vi "Process.vi"(8 "error in":errorcluster, 11 "SystemController":refnum<class "SystemController.lvclass">) -> (0 "error out":errorcluster, 3 "SystemController out":refnum<class "SystemController.lvclass">)   [LabVIEW 2017, in "SystemController.lvclass"]
doc: "---------------------------------------------------------------\nJKI State Machine Objects™\nhttp://jki.net/state-machine-objects/\nCopyright (C) 2005-2015, JKI <info@jki.net>\nALL RIGHTS RESERVEDJKI State Machine Objects (SMO) 1.0.0.5\nJKI - JKI\nCopyright (c) 2016, JKI"
uses:
  SystemController.lvclass
  C:/Program Files (x86)/National Instruments/LabVIEW 2017/vi.lib/JKI/JKI SMO/SMO/SMO.lvclass
  <vilib>/JKI/JKI SMO/SMO/Typedefs/Parent Call--Enum.ctl
  ImageFacialDetection_class/FindFaces_IMAQ.vi
  ImageFacialDetection_class/FindEyes_IMAQ.vi
  <vilib>/JKI/JKI SMO/SMO/SMO.lvclass
  Camera/Camera_class/Camera.lvclass
  ImageFacialDetection_class/ImageFacialDetection.lvclass
panel:
  out "Image":T1(plugin-control)
  out "Connected":bool
  # "For instructions on how to use the JKI State Machine Objects, examples and video tutorials, visit:\nhttp://jki.net/state-machine-objects/\n\nJKI State Machine Objects™\nhttp://jki.net/state-machine-objects/\nCopyright (C) 2005-2015, JKI <info@jki.net>\nALL RIGHTS RESERVED"
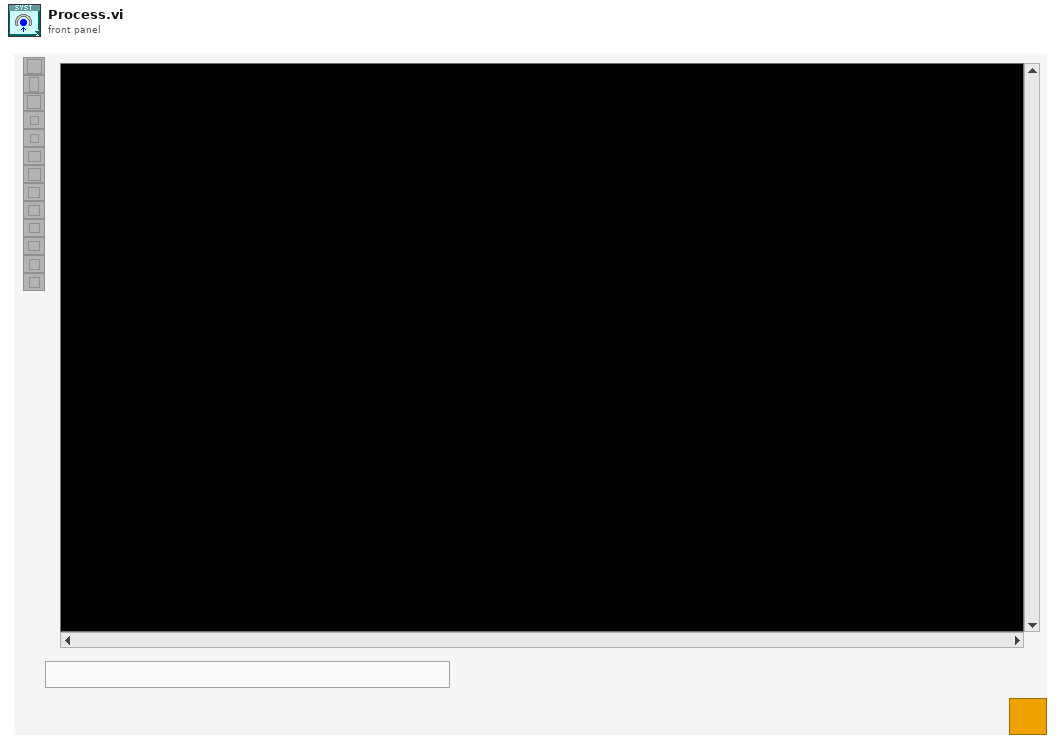
[diagram p1: front panel]
types:
  T1 = typedef "IMAQ Image.ctl" = refnum<image>
  T2 = typedef "SMO.lvclass/Parent Call--Enum.ctl" = enum16{"Allows parent to run", "Does not request parent to run"}
  T3 = enum32{"invalid app kind", "Development System", "Run Time System", "Student Edition", "Embedded LabVIEW", "Evaluation", "Custom"}
  T4 = enum32{"Invalid", "Standard", "Closed", "Hidden", "Minimized", "Maximized"}
  T5 = typedef "SystemController.lvclass/Configuration--Cluster.ctl" = cluster{"Camera":T6, "Find Eyes":bool, "Acquisition Rate (ms)":i32, "Image Buffer Length":i32}
  T6 = typedef "SystemController.lvclass/CameraConfig--Cluster.ctl" = cluster{"Simulate Camera":bool, "IMAQ Camera":T7, "Simulated Image Folder":path}
  T7 = typedef "Camera_IMAQdx.lvclass/Configuration--Cluster.ctl" = cluster{"Camera Interface Name":string, "Number of Buffers":u32, "Image Name":string, "Image Type":T8}
  T8 = typedef "Image Type" = u32
  T9 = typedef "SystemController.lvclass/Dependencies--Cluster.ctl" = cluster{"Camera":refnum<class "Camera.lvclass">, "ImageFacialDetection":refnum<class "ImageFacialDetection.lvclass">}
  T10 = cluster{"Core":cluster{"Current VI Reference":refnum<vi>, "Close Panel on Exit?":bool, "error":errorcluster}, "Self Reference":refnum<class "SystemController.lvclass">, "Dependencies":T9, "Find Eyes":bool, "Camera Connected":bool, "New Image":T1}
  T11 = cluster{"Current VI Reference":refnum<vi>, "Close Panel on Exit?":bool, "error":errorcluster}
  T12 = typedef "SMO.lvclass/Protected Events.ctl" = cluster{"StopProcesses":refnum<user-event>, "AbortProcesses":refnum<user-event>, "Config Changed":refnum<user-event>, "Dependency":refnum<user-event>}
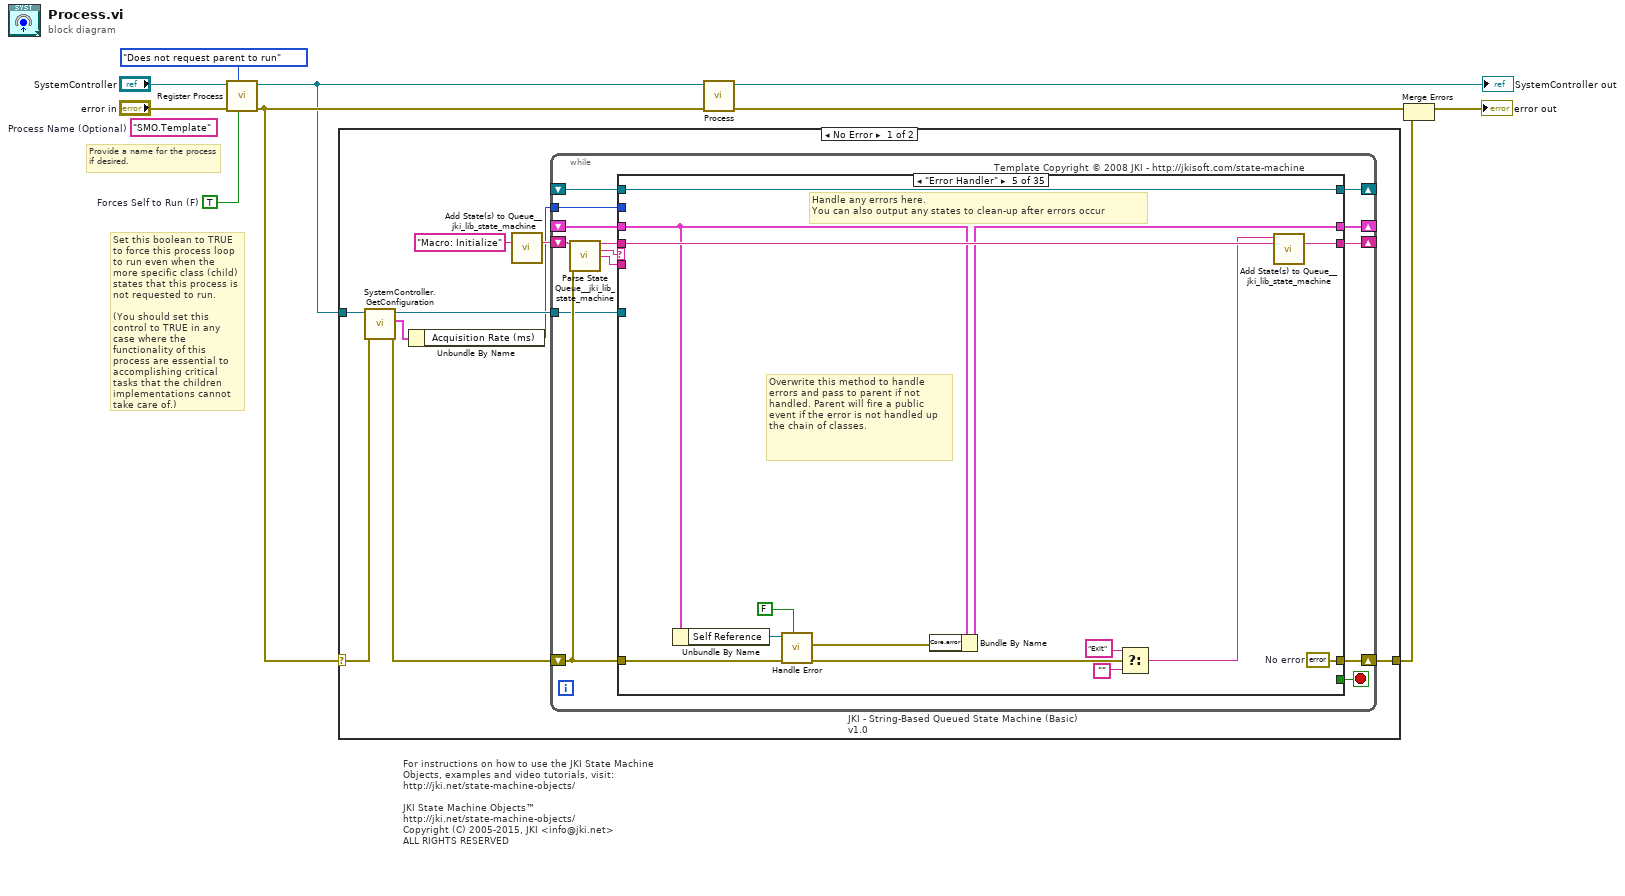
[diagram p0: block diagram]
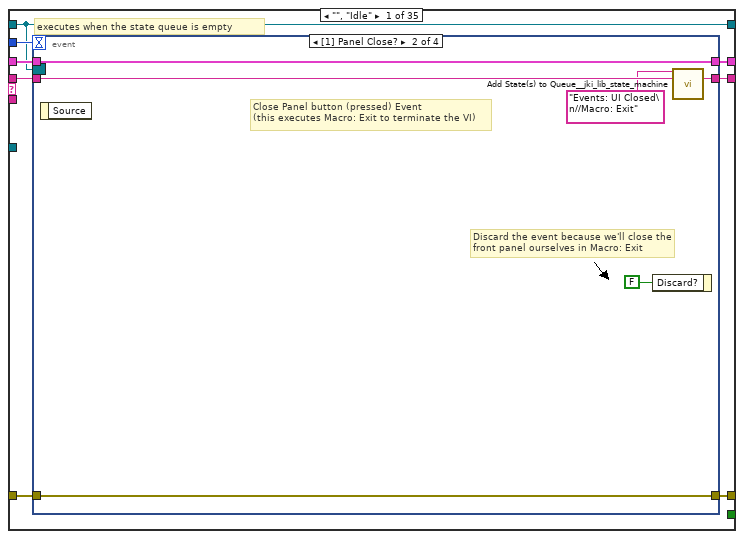
[diagram p2: hidden frame]
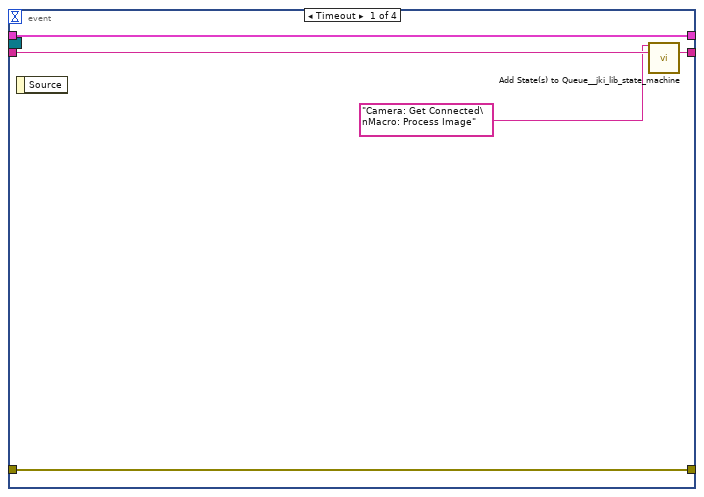
[diagram p3: hidden frame]
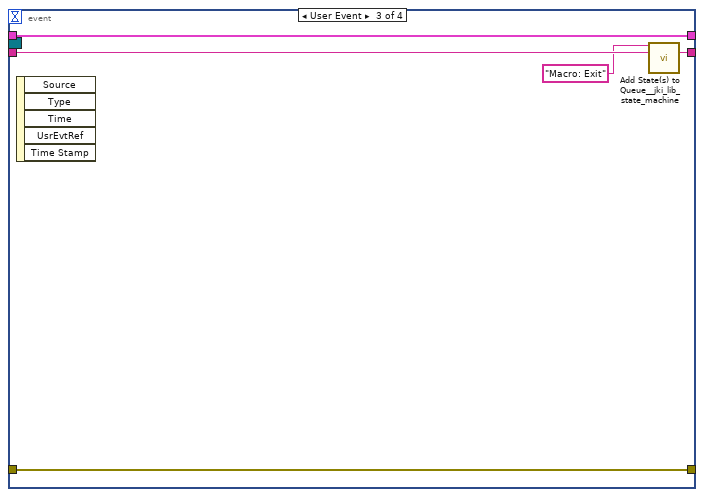
[diagram p4: hidden frame]
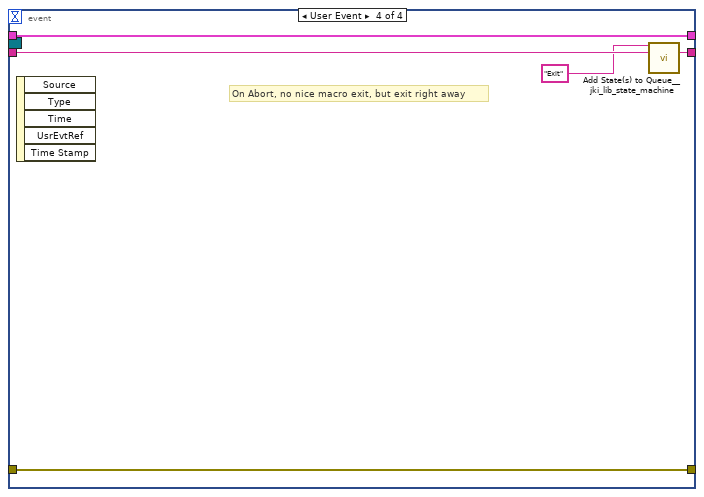
[diagram p5: hidden frame]
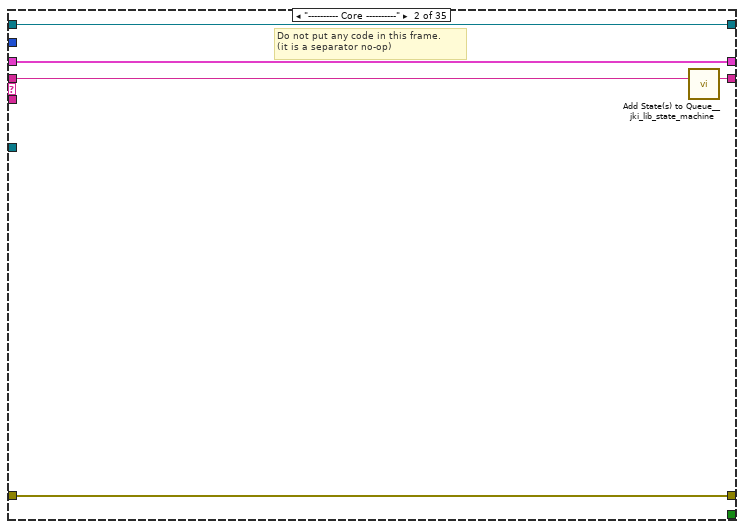
[diagram p6: hidden frame]
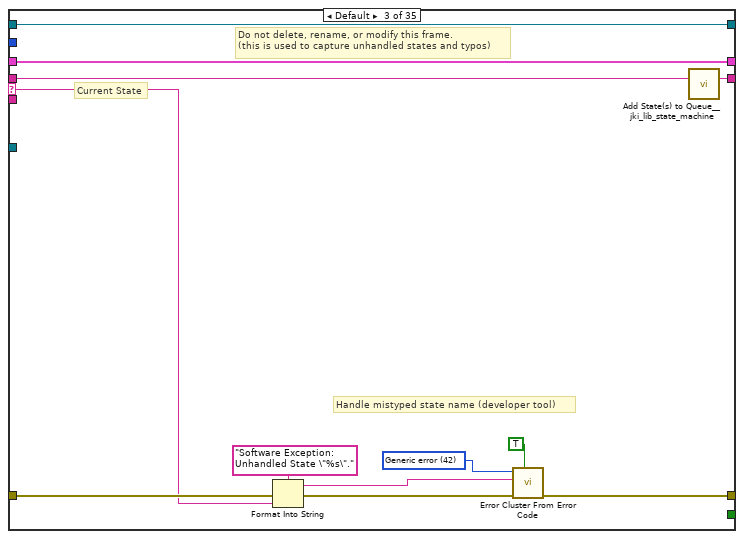
[diagram p7: hidden frame]
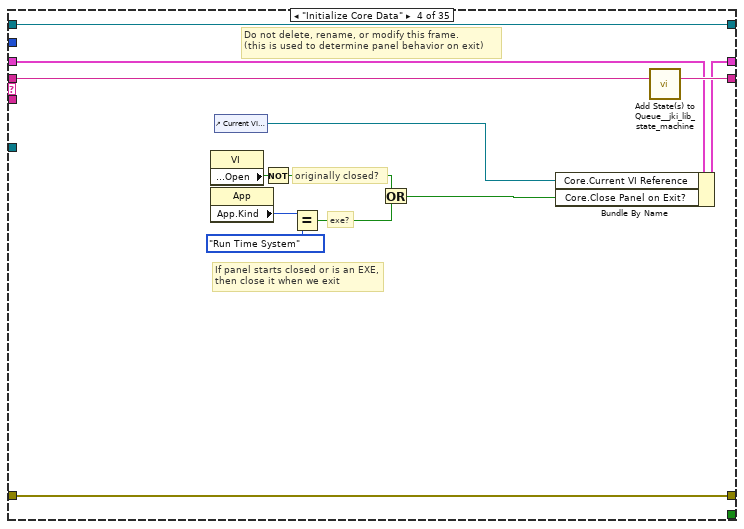
[diagram p8: hidden frame]
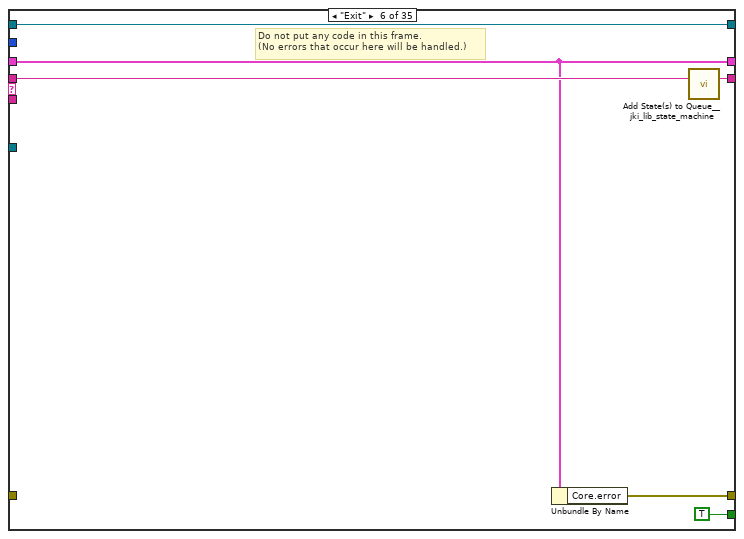
[diagram p9: hidden frame]
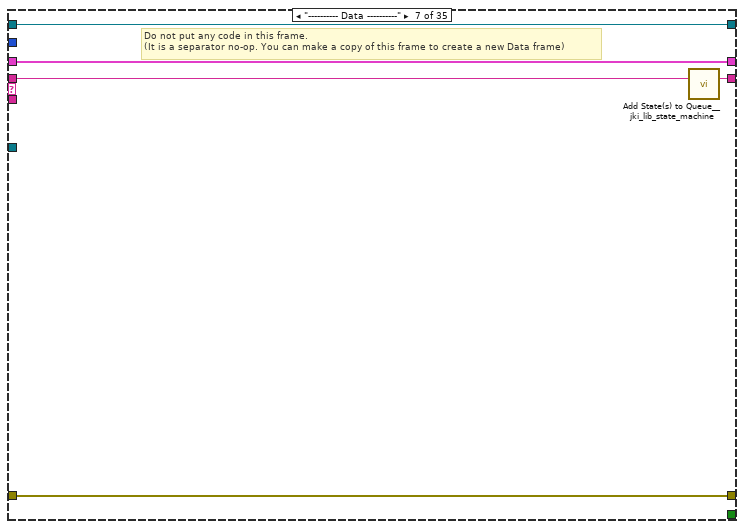
[diagram p10: hidden frame]
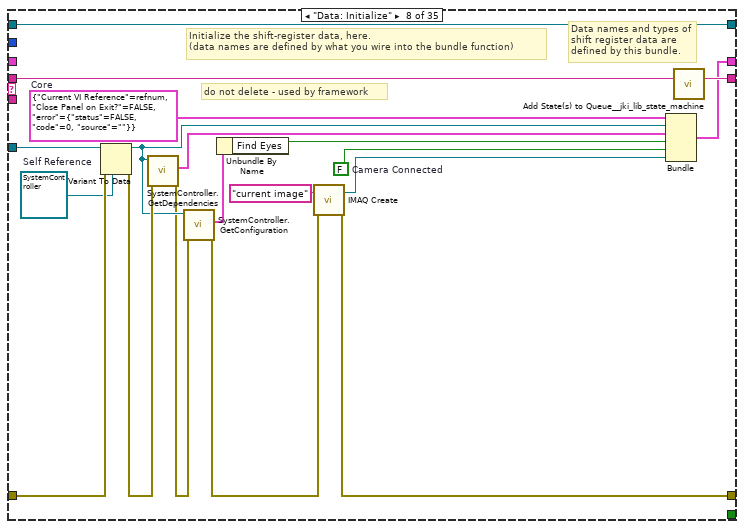
[diagram p11: hidden frame]
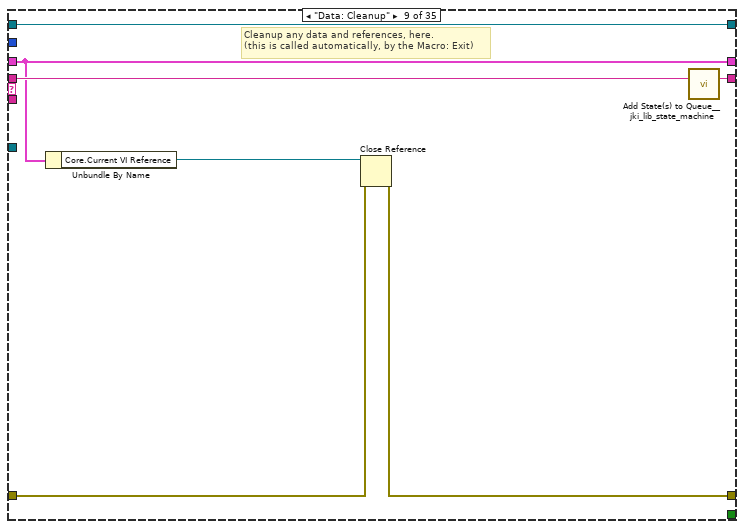
[diagram p12: hidden frame]
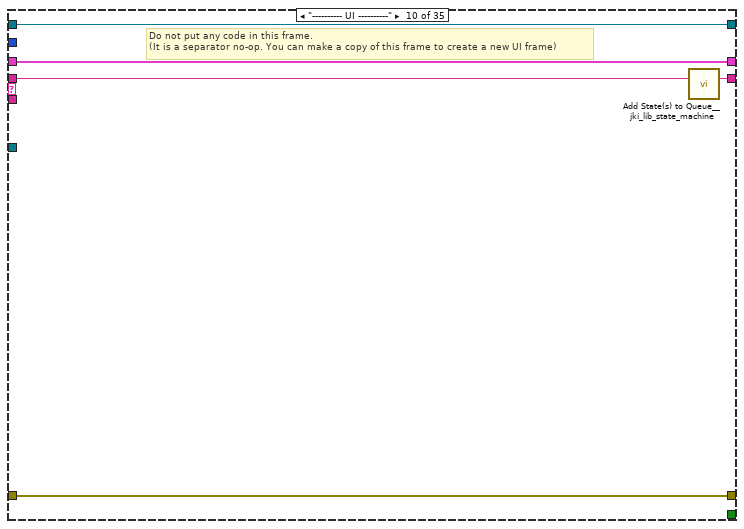
[diagram p13: hidden frame]
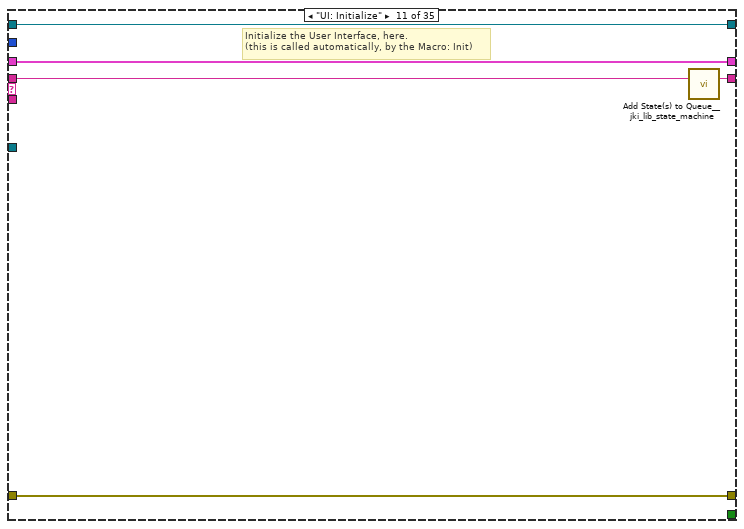
[diagram p14: hidden frame]
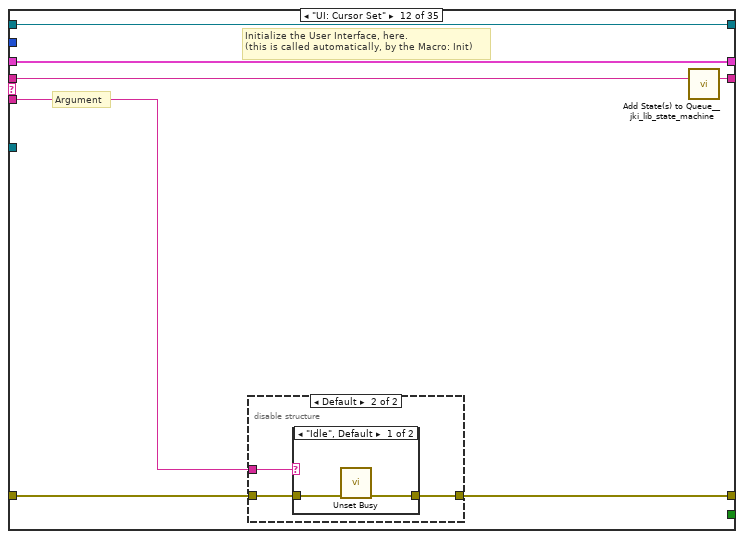
[diagram p15: hidden frame]
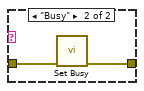
[diagram p17: hidden frame]
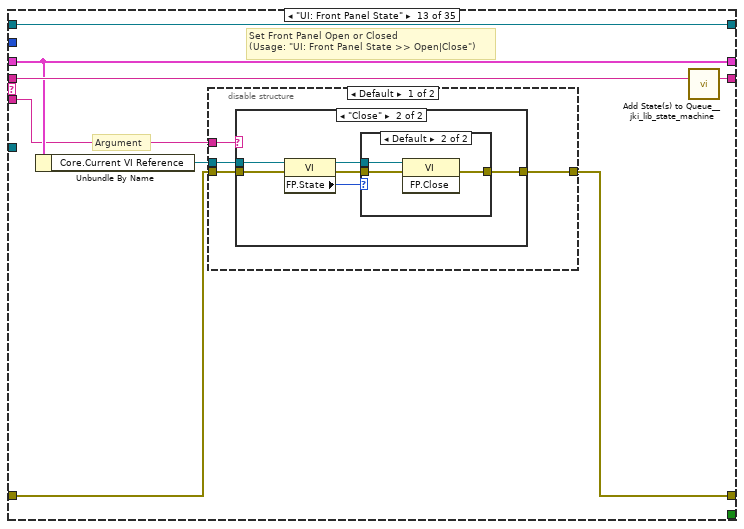
[diagram p18: hidden frame]
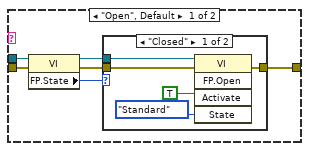
[diagram p19: hidden frame]
diagram:
  w1 = TRUE  # Forces Self to Run (F)
  (unwired) "SMO.Template"  # Process Name (Optional)
  # "Provide a name for the process\nif desired."
  # "Set this boolean to TRUE to force this process loop to run even when the more specific class (child) states that this process is not requested to run.\n\n(You should set this control to TRUE in any case where the functionality of this process are essential to accomplishing critical tasks that the children implementations cannot take care of.)"
  # "For instructions on how to use the JKI State Machine Objects, examples and video tutorials, visit:\nhttp://jki.net/state-machine-objects/\n\nJKI State Machine Objects™\nhttp://jki.net/state-machine-objects/\nCopyright (C) 2005-2015, JKI <info@jki.net>\nALL RIGHTS RESERVED"
  n1 = call <vilib>:"Register Process.vi"("Forces Self to Run (F)"=w1, "Parent Call"=Parent_Call--Enum."Does not request parent to run", "error in (no error)"="error in", "SMO"="SystemController") -> ("error out"=w7:errorcluster, "SMO out"=w6:refnum<class "SystemController.lvclass">)  [unwired: 6 in]
  n2 = case shown="No Error" w7 {
    selector: w7 -> [w12 w383]
    tunnel: w6 -> [w17 _]
    tunnel: [w16 w383] -> w3
    frame No Error {
      n3 = call "SystemController.GetConfiguration.vi"("error in (no error)"=w12, "SystemController"=w17) -> ("error out"=w11:errorcluster, "Configuration"=w14:T5, "SystemController out"=w15:refnum<class "SystemController.lvclass">)  [unwired: 7 in]
      n4 = Unbundle By Name(w14) -> ("Acquisition Rate (ms)"=w13:i32)
      n5 = call <vilib>:"Add State(s) to Queue__jki_lib_state_machine.vi"("State(s) in (\"\")"="Macro: Initialize") -> ("States Out"=w19:string)  [unwired: 14 in]
      n6 = while "JKI - String-Based Queued State Machine (Basic) v1.0" {
        shift-right: [w26] -> _
        shift-left: _ -> [w25]
        shift-right: [w29] -> w16
        shift-left: w11 -> [w24]
        shift-right: [w28] -> _
        shift-left: w19 -> [w30]
        tunnel: w15 -> [w23]
        shift-right: [w22] -> _
        shift-left: _ -> [w21]
        tunnel: w13 -> [w20]
        stop <- w27 stop-if-true
        # "Template Copyright © 2008 JKI - http://jkisoft.com/state-machine"
        n7 = call <vilib>:"Parse State Queue__jki_lib_state_machine.vi"("State Queue"=w30, "Error In (no error)"=w24) -> ("Remaining States"=w32:string, "Current State"=w33:string, "Arguments"=w31:string)  [unwired: 11 in]
        n8 = case shown="\"Error Handler\"" w33 {
          selector: w33 -> [_ _ w69 _ _ _ _ _ _ _ _ _ _ _ _ _ _ _ _ _ _ _ _ _ _ _ _ _ _ _ _ _ _ _ _]
          tunnel: w32 -> [w41 w67 w73 w92 w106 w112 w117 w136 w143 w148 w153 w160 w176 w208 w223 w232 w246 w251 w262 w267 w274 w284 w290 w295 w302 w309 w316 w323 w335 w344 w349 w359 w369 w374 w382]
          tunnel: w31 -> [_ _ _ _ _ _ _ _ _ _ _ w154 w170 _ _ _ _ _ _ _ _ _ _ _ _ _ _ _ _ _ _ _ _ _ _]
          tunnel: w25 -> [w39 w64 w71 w83 w95 w108 w114 _ w138 w145 w151 w158 w172 w205 w219 w228 w237 w248 w259 w264 w271 w282 w288 w293 w299 w306 w313 w320 w330 w338 w347 w352 w362 w372 w379]
          tunnel: [w38 w65 w75 w89 w97 w107 w115 w118 w139 w146 w150 w155 w173 w206 w221 w230 w244 w249 w253 w265 w268 w275 w286 w291 w296 w303 w310 w317 w324 w339 w345 w353 w363 w370 w376] -> w29
          tunnel: w24 -> [w37 w65 w74 w89 w102 _ w115 w133 w140 w146 w150 w156 w174 w206 w221 w230 w244 w249 w254 w265 w269 w278 w286 w291 w297 w304 w311 w318 w331 w340 w345 w354 w364 w370 w377]
          tunnel: [w40 w66 w72 w91 w105 w111 w116 w135 w142 w147 w152 w159 w175 w207 w222 w231 w245 w250 w261 w266 w273 w283 w289 w294 w301 w308 w315 w322 w334 w343 w348 w358 w368 w373 w381] -> w28
          tunnel: [_ _ _ _ _ TRUE _ _ _ _ _ _ _ _ _ _ _ _ _ _ _ _ _ _ _ _ _ _ _ _ _ _ _ _ _] -> w27
          tunnel: [w36 w64 w71 w90 w94 w108 w114 w134 w138 w145 w151 w158 w172 w205 w219 w228 w237 w248 w259 w264 w271 w282 w288 w293 w299 w306 w313 w320 w329 w337 w347 w351 w361 w372 w379] -> w26
          tunnel: w20 -> [w35 _ _ _ _ _ _ _ _ _ _ _ _ _ _ _ _ _ _ _ _ _ _ _ _ _ _ _ _ _ _ _ _ _ _]
          tunnel: w23 -> [_ _ _ _ _ _ _ w131 _ _ _ _ _ _ _ _ _ _ _ _ _ _ _ _ _ _ _ _ _ _ _ _ _ _ _]
          tunnel: [w34 w63 w68 w80 w104 w109 w113 w130 w137 w144 w149 w157 w169 w204 w220 w229 w238 w247 w260 w263 w272 w281 w287 w292 w300 w307 w314 w321 w333 w342 w346 w357 w367 w371 w380] -> w22
          tunnel: w21 -> [w34 w63 w68 w80 w104 w109 w113 w130 w137 w144 w149 w157 w169 w204 w220 w229 w238 w247 w260 w263 w272 _ w287 w292 w300 w307 w314 w321 w333 w342 w346 w357 w367 w371 w380]
          frame "", "Idle" {
            # "executes when the state queue is empty"
            n9 = event shown="[1] Panel Close?" {
              selector: w34 -> [_ _ _ _]
              dyn-events: _ -> [_ _ _ _]
              timeout: w35 -> [_ _ _ _]
              tunnel: w41 -> [w46 w52 w57 w62]
              tunnel: [w45 w51 w56 w61] -> w40
              tunnel: w39 -> [w43 w49 w54 w59]
              tunnel: [w44 w50 w55 w60] -> w38
              tunnel: w37 -> [w44 w50 w55 w60]
              tunnel: [w43 w49 w54 w59] -> w36
              event Timeout {
                n10 = event-data() -> ()  [unwired: 1 in, 1 out]
                n11 = call <vilib>:"Add State(s) to Queue__jki_lib_state_machine.vi"("State(s) in Front (\"\")"="Camera: Get Connected\nMacro: Process Image", "State(s) in (\"\")"=w46) -> ("States Out"=w45:string)  [unwired: 13 in]
              }
              event Panel Close? {
                # "Discard the event because we'll close the front panel ourselves in Macro: Exit"
                # "Close Panel button (pressed) Event\n(this executes Macro: Exit to terminate the VI)"
                n12 = event-data() -> ()  [unwired: 1 in, 1 out]
                n13 = event-data("Discard?"=FALSE) -> ()  [unwired: 1 in, 1 out]
                n14 = call <vilib>:"Add State(s) to Queue__jki_lib_state_machine.vi"("State(s) in Front (\"\")"="Events: UI Closed\n//Macro: Exit", "State(s) in (\"\")"=w52) -> ("States Out"=w51:string)  [unwired: 13 in]
              }
              event User Event {
                n15 = event-data() -> ()  [unwired: 1 in, 5 out]
                n16 = call <vilib>:"Add State(s) to Queue__jki_lib_state_machine.vi"("State(s) in Front (\"\")"="Macro: Exit", "State(s) in (\"\")"=w57) -> ("States Out"=w56:string)  [unwired: 13 in]
              }
              event User Event {
                # "On Abort, no nice macro exit, but exit right away"
                n17 = event-data() -> ()  [unwired: 1 in, 5 out]
                n18 = call <vilib>:"Add State(s) to Queue__jki_lib_state_machine.vi"("State(s) in Front (\"\")"="Exit", "State(s) in (\"\")"=w62) -> ("States Out"=w61:string)  [unwired: 13 in]
              }
            }
          }
          frame "---------- Core ----------" {
            # "Do not put any code in this frame.\n(it is a separator no-op)"
            n19 = call <vilib>:"Add State(s) to Queue__jki_lib_state_machine.vi"("State(s) in (\"\")"=w67) -> ("States Out"=w66:string)  [unwired: 14 in]
          }
          frame Default {
            w78 = 42 items=["No error", "Argument error", "Memory is full", "Out of zone", "End of file", "File already open", "Generic file I/O error", "File not found", "File permission error", "Disk is full", "Duplicate path", "Too many files open", "System feature not enabled", "Resource file not found", "Cannot add resource", "Resource not found", "Image not found", "Image memory error", "Pen does not exist", "Config type invalid", "Config token not found", "Config parse error", "Config memory error", "Bad external code format", "Bad external code offset", "External code not present", "Null window", "Destroy window error", "Null menu", "Print aborted", "Bad print record", "Print driver error", "Windows error during printing", "Memory error during printing", "Print dialog error", "Generic print error", "Invalid device refnum", "Device not found", "Device parameter error", "Device unit error", "Cannot open device", "Device call aborted", "Generic error", "Cancelled by user", "Object ID too low", "Object ID too high", "Object not in heap", "Unknown heap", "Unknown object (invalid DefProc)", "Unknown object (DefProc not in table)", "Message out of range", "Invalid (null) method", "Unknown message", "Manager call not supported", "Bad address", "Network operation in progress", "Network operation timed out", "Connection is busy", "Network attribute not supported", "Network error", "Address in use", "System out of memory", "Connection aborted", "Connection refused", "Not connected", "Already connected", "Connection closed", "Initialization error (interapplication manager)", "Bad occurrence", "Wait on unbound occurrence handler", "Occurrence queue overflow", "Datalog type conflict", "Unused", "Unrecognized type (interapplication manager)", "Memory corrupt", "Failed to make temporary DLL", "Old CIN version", "Drag socket not found", "Failed to load drop-object", "Failed to register OLE object", "Failed to release OLE object", "Format specifier type mismatch", "Unknown format specifier", "Too few format specifiers", "Too many format specifiers", "Scan failed", "Newer CIN version", "Error converting to variant", "Runtime menu error", "Password tampered", "Variant attribute not found", "Incompatible variant data type", "Event data is not available", "Event Store is not present", "Occurrence is not found", "Event Queue is not created", "Event info is not available", "Refnum passed is NULL", "Error retrieving Class GUID", "Error retrieving CoClass GUID", "Error retrieving TypeLib GUID.", "Bad built application magic bytes.", "Specific driver is different from the specific driver associated with the Logical Name.", "There is no session opened to the class driver.", "Max Error", "MAX - Error with config objects", "MAX - Error loading configuration", "MAX - Group not supported"]
            # "Current State"
            # "Do not delete, rename, or modify this frame.\n(this is used to capture unhandled states and typos)"
            # "Handle mistyped state name (developer tool)"
            n20 = Format Into String(format string="Software Exception: Unhandled State \"%s\"." ("message"), error in=w74, w69) -> (resulting string=w77:string, error out=w76:errorcluster)  [unwired: 1 in]
            n21 = call <vilib>:"Error Cluster From Error Code.vi"("show call chain? (False)"=TRUE, "error in (no error)"=w76, "error message (\"\")"=w77, "error code (0)"=w78) -> ("error out"=w75:errorcluster)  [unwired: 5 in]
            n22 = call <vilib>:"Add State(s) to Queue__jki_lib_state_machine.vi"("State(s) in (\"\")"=w73) -> ("States Out"=w72:string)  [unwired: 14 in]
          }
          frame "Initialize Core Data" {
            # "Do not delete, rename, or modify this frame.\n(this is used to determine panel behavior on exit)"
            # "originally closed?"
            # "exe?"
            # "If panel starts closed or is an EXE, then close it when we exit"
            n23 = property class="VI"() -> ("Front Panel.Open"=w88:bool)  [unwired: 2 in, 2 out]
            n24 = property class="App"() -> ("App.Kind"=w87:T3)  [unwired: 2 in, 2 out]
            n25 = control-ref of="Current VI Reference"() -> (w81:refnum<vi>)
            n26 = Not(x=w88) -> (.not. x?=w85:bool)
            n27 = Equal?(x=w87, y=T3."Run Time System" ("Application:Kind")) -> (x = y?=w84:bool)
            n28 = Or(x=w85, y=w84) -> (x .or. y?=w82:bool)
            n29 = Bundle By Name(cluster=w83, "Core.Current VI Reference"=w81, "Core.Close Panel on Exit?"=w82) -> (w90:T10)
            n30 = call <vilib>:"Add State(s) to Queue__jki_lib_state_machine.vi"("State(s) in (\"\")"=w92) -> ("States Out"=w91:string)  [unwired: 14 in]
          }
          frame "Error Handler" {
            w97 = errorcluster {"status"=FALSE, "code"=0, "source"=""}  # No error
            # "Overwrite this method to handle errors and pass to parent if not handled. Parent will fire a public event if the error is not handled up the chain of classes."
            # "Handle any errors here.\nYou can also output any states to clean-up after errors occur"
            n31 = Unbundle By Name(w95) -> ("Self Reference"=w103:refnum<class "SystemController.lvclass">)
            n32 = call-dynamic "Handle Error.vi"("Stop on Unhandled Error (T)"=FALSE, "error in"=w102, "SMO"=w103) -> ("handling error"=w98:errorcluster, "Unhandled error"=w96:errorcluster)  [unwired: 6 in, 1 out]
            n33 = Bundle By Name(cluster=w95, "Core.error"=w96) -> (w94:T10)
            n34 = Select(t="Exit", s=w98, f="") -> (s? t:f=w99:string)
            n35 = call <vilib>:"Add State(s) to Queue__jki_lib_state_machine.vi"("State(s) in Front (\"\")"=w99, "State(s) in (\"\")"=w106) -> ("States Out"=w105:string)  [unwired: 13 in]
          }
          frame "Exit" {
            # "Do not put any code in this frame.\n(No errors that occur here will be handled.)"
            n36 = Unbundle By Name(w108) -> ("Core.error"=w107:errorcluster)
            n37 = call <vilib>:"Add State(s) to Queue__jki_lib_state_machine.vi"("State(s) in (\"\")"=w112) -> ("States Out"=w111:string)  [unwired: 14 in]
          }
          frame "---------- Data ----------" {
            # "Do not put any code in this frame.\n(It is a separator no-op. You can make a copy of this frame to create a new Data frame)"
            n38 = call <vilib>:"Add State(s) to Queue__jki_lib_state_machine.vi"("State(s) in (\"\")"=w117) -> ("States Out"=w116:string)  [unwired: 14 in]
          }
          frame "Data: Initialize" {
            w122 = FALSE  # Camera Connected
            w129 = T11 {"Current VI Reference"=refnum, "Close Panel on Exit?"=FALSE, "error"={"status"=FALSE, "code"=0, "source"=""}}  # Core
            w132 = refnum<class "SystemController.lvclass"> refnum  # Self Reference
            # "do not delete - used by framework"
            # "Data names and types of shift register data are defined by this bundle."
            # "Initialize the shift-register data, here.\n(data names are defined by what you wire into the bundle function)"
            n39 = Variant To Data(error in=w133, type=w132, Variant=w131) -> (data=w126:refnum<class "SystemController.lvclass">, error out=w127:errorcluster)
            n40 = call "SystemController.GetDependencies.vi"("error in (no error)"=w127, "SystemController"=w126) -> ("error out"=w125:errorcluster, "Dependencies"=w128:T9)  [unwired: 7 in, 1 out]
            n41 = call "SystemController.GetConfiguration.vi"("error in (no error)"=w125, "SystemController"=w126) -> ("error out"=w119:errorcluster, "Configuration"=w124:T5)  [unwired: 7 in, 1 out]
            n42 = Unbundle By Name(w124) -> ("Find Eyes"=w123:bool)
            n43 = call "IMAQ Create"("Image Name"="current image", "error in (no error)"=w119) -> ("New Image"=w120:T1, "error out"=w118:errorcluster)  [unwired: 3 in]
            n44 = Bundle("Core"=w129, "Self Reference"=w126, "Dependencies"=w128, "Find Eyes"=w123, "Camera Connected"=w122, "New Image"=w120) -> (w134:T10)  [unwired: 1 in]
            n45 = call <vilib>:"Add State(s) to Queue__jki_lib_state_machine.vi"("State(s) in (\"\")"=w136) -> ("States Out"=w135:string)  [unwired: 14 in]
          }
          frame "Data: Cleanup" {
            # "Cleanup any data and references, here.\n(this is called automatically, by the Macro: Exit)"
            n46 = Unbundle By Name(w138) -> ("Core.Current VI Reference"=w141:refnum<vi>)
            n47 = Close Reference(reference=w141, error in (no error)=w140) -> (error out=w139:errorcluster)
            n48 = call <vilib>:"Add State(s) to Queue__jki_lib_state_machine.vi"("State(s) in (\"\")"=w143) -> ("States Out"=w142:string)  [unwired: 14 in]
          }
          frame "---------- UI ----------" {
            # "Do not put any code in this frame.\n(It is a separator no-op. You can make a copy of this frame to create a new UI frame)"
            n49 = call <vilib>:"Add State(s) to Queue__jki_lib_state_machine.vi"("State(s) in (\"\")"=w148) -> ("States Out"=w147:string)  [unwired: 14 in]
          }
          frame "UI: Initialize" {
            # "Initialize the User Interface, here.\n(this is called automatically, by the Macro: Init)"
            n50 = call <vilib>:"Add State(s) to Queue__jki_lib_state_machine.vi"("State(s) in (\"\")"=w153) -> ("States Out"=w152:string)  [unwired: 14 in]
          }
          frame "UI: Cursor Set" {
            # "Argument"
            # "Initialize the User Interface, here.\n(this is called automatically, by the Macro: Init)"
            n51 = disable-structure shown="Default" {
              disable-tunnel: w156 -> [w161 w164]
              disable-tunnel: [w161 w163] -> w155
              disable-tunnel: w154 -> [_ w162]
              frame condition #0 {
              }
              frame condition #1 (active) {
                n52 = case shown="\"Idle\", Default" w162 {
                  tunnel: w164 -> [w166 w168]
                  tunnel: [w165 w167] -> w163
                  frame "Idle", Default {
                    n53 = call <vilib>:"Unset Busy.vi"("error in (no error)"=w166) -> ("error out"=w165:errorcluster)  [unwired: 10 in]
                  }
                  frame "Busy" {
                    n54 = call <vilib>:"Set Busy.vi"("error in (no error)"=w168) -> ("error out"=w167:errorcluster)  [unwired: 9 in, 1 out]
                  }
                }
              }
            }
            n55 = call <vilib>:"Add State(s) to Queue__jki_lib_state_machine.vi"("State(s) in (\"\")"=w160) -> ("States Out"=w159:string)  [unwired: 14 in]
          }
          frame "UI: Front Panel State" {
            # "Argument"
            # "Set Front Panel Open or Closed\n(Usage: \"UI: Front Panel State >> Open|Close\")"
            n56 = Unbundle By Name(w172) -> ("Core.Current VI Reference"=w171:refnum<vi>)
            n57 = disable-structure shown="Default" {
              disable-tunnel: w174 -> [w180 w203]
              disable-tunnel: [w179 w203] -> w173
              disable-tunnel: w171 -> [w178 _]
              disable-tunnel: w170 -> [w177 _]
              frame condition #0 (active) {
                n58 = case shown="\"Close\"" w177 {
                  tunnel: w180 -> [w184 w197]
                  tunnel: [w186 w198] -> w179
                  tunnel: w178 -> [w185 w195]
                  frame "Open", Default {
                    n59 = property class="VI"(reference=w185, error in=w184) -> (reference out=w182:refnum<vi>, error out=w183:errorcluster, "FP.State"=w181:T4)
                    n60 = case shown="\"Closed\"" w181 {
                      tunnel: [w189 w192] -> w186
                      tunnel: w183 -> [w188 w192]
                      tunnel: w182 -> [w187 _]
                      frame "Closed" {
                        n61 = invoke class="VI" method="FP.Open"(reference=w187, error in=w188, "Activate"=TRUE, "State"=T4."Standard") -> (error out=w189:errorcluster)  [unwired: 1 in, 4 out]
                      }
                      frame Default {
                      }
                    }
                  }
                  frame "Close" {
                    n62 = property class="VI"(reference=w195, error in=w197) -> (reference out=w194:refnum<vi>, error out=w196:errorcluster, "FP.State"=w193:T4)
                    n63 = case shown="Default" w193 {
                      tunnel: [w199 w202] -> w198
                      tunnel: w196 -> [w199 w201]
                      tunnel: w194 -> [_ w200]
                      frame "Invalid", "Closed" {
                      }
                      frame Default {
                        n64 = invoke class="VI" method="FP.Close"(reference=w200, error in=w201) -> (error out=w202:errorcluster)  [unwired: 1 in, 2 out]
                      }
                    }
                  }
                }
              }
              frame condition #1 {
              }
            }
            n65 = call <vilib>:"Add State(s) to Queue__jki_lib_state_machine.vi"("State(s) in (\"\")"=w176) -> ("States Out"=w175:string)  [unwired: 14 in]
          }
          frame "---------- Macro ----------" {
            # "Do not put any code in this frame.\n(It is a separator no-op. You can make a copy of this frame to create a new Macro frame)"
            n66 = call <vilib>:"Add State(s) to Queue__jki_lib_state_machine.vi"("State(s) in (\"\")"=w208) -> ("States Out"=w207:string)  [unwired: 14 in]
          }
          frame "Macro: Process Image" {
            # "If Connected (\nGrab\nFind Faces\nIf (find eyes = T) Find Eyes\nSet Image\n)"
            n67 = Unbundle By Name(w219) -> ("Find Eyes"=w216:bool, "Camera Connected"=w212:bool)
            n68 = Select(t="Facial Recognition: Find Eyes", s=w216, f="") -> (s? t:f=w215:string)
            n69 = call <vilib>:"Add State(s) to Queue__jki_lib_state_machine.vi"("State(s) in Front (\"\")"="Camera: Grab\nFacial Recognition: Find Faces", "State(s) in (\"\")"=w215, "State(s) at Back (\"\")"="Image: Set") -> ("States Out"=w211:string)  [unwired: 12 in]
            n70 = Select(t=w211, s=w212, f="") -> (s? t:f=w209:string)
            n71 = call <vilib>:"Add State(s) to Queue__jki_lib_state_machine.vi"("State(s) in Front (\"\")"=w209, "State(s) in (\"\")"=w223) -> ("States Out"=w222:string)  [unwired: 13 in]
          }
          frame "Macro: Initialize" {
            w226 = "Camera: Connect\nCamera: Start Acquisition\nUI: Initialize\nUI: Front Panel State >> Open"  # Camera: Connect Camera: Start Acquisition UI: Initialize UI: Front Panel State >> Open
            # "Initialization Macro\n(This is called once, when the VI starts)"
            n72 = call <vilib>:"Add State(s) to Queue__jki_lib_state_machine.vi"("State(s) in Front (\"\")"="Data: Initialize\nInitialize Core Data\nEvents: Register", "State(s) in (\"\")"="Process: Sync", "State(s) at Back (\"\")"=w226) -> ("States Out"=w225:string)  [unwired: 12 in]
            n73 = call <vilib>:"Add State(s) to Queue__jki_lib_state_machine.vi"("State(s) in Front (\"\")"=w225, "State(s) in (\"\")"=w232) -> ("States Out"=w231:string)  [unwired: 13 in]
          }
          frame "Macro: Exit" {
            # "Exit Macro\n(This is called once, when the VI exits)"
            n74 = Unbundle By Name(w237) -> ("Core.Close Panel on Exit?"=w243:bool)
            n75 = Select(t="UI: Front Panel State >> Close", s=w243, f="") -> (s? t:f=w240:string)
            n76 = call <vilib>:"Add State(s) to Queue__jki_lib_state_machine.vi"("State(s) in Front (\"\")"="Camera: Stop Acquisition\nCamera: Disconnect\nData: Cleanup\nEvents: Unregister", "State(s) in (\"\")"="Process: Sync", "State(s) at Back (\"\")"="Exit") -> ("States Out"=w234:string)  [unwired: 12 in]
            n77 = call <vilib>:"Add State(s) to Queue__jki_lib_state_machine.vi"("State(s) in (\"\")"=w240, "State(s) at Back (\"\")"=w234) -> ("States Out"=w239:string)  [unwired: 13 in]
            n78 = call <vilib>:"Add State(s) to Queue__jki_lib_state_machine.vi"("State(s) in Front (\"\")"=w239, "State(s) in (\"\")"=w246) -> ("States Out"=w245:string)  [unwired: 13 in]
          }
          frame "---------- Process ----------" {
            # "Template Separator\n(You can make a copy of, or modify, this frame)"
            n79 = call <vilib>:"Add State(s) to Queue__jki_lib_state_machine.vi"("State(s) in (\"\")"=w251) -> ("States Out"=w250:string)  [unwired: 14 in]
          }
          frame "Process: Sync" {
            n80 = Unbundle By Name(w259) -> ("Self Reference"=w255:refnum<class "SystemController.lvclass">)
            n81 = call <vilib>:"WaitOnProcessSync.vi"("error in (no error)"=w254, "SMO"=w255) -> ("error out"=w253:errorcluster, "Don't run?"=w258:bool)  [unwired: 7 in, 1 out]
            n82 = Select(t="Data: Cleanup\nEvents: Unregister\nExit", s=w258, f="") -> (s? t:f=w252:string)
            n83 = call <vilib>:"Add State(s) to Queue__jki_lib_state_machine.vi"("State(s) in Front (\"\")"=w252, "State(s) in (\"\")"=w262) -> ("States Out"=w261:string)  [unwired: 13 in]
          }
          frame "---------- Events ----------" {
            # "Template Separator\n(You can make a copy of, or modify, this frame)"
            n84 = call <vilib>:"Add State(s) to Queue__jki_lib_state_machine.vi"("State(s) in (\"\")"=w267) -> ("States Out"=w266:string)  [unwired: 14 in]
          }
          frame "Events: UI Closed" {
            # "Notidy launcher that the UI was closed"
            n85 = Unbundle By Name(w271) -> ("Self Reference"=w270:refnum<class "SystemController.lvclass">)
            n86 = call "SystemController.UIClosed.vi"("error in (no error)"=w269, "SystemController"=w270) -> ("error out"=w268:errorcluster)  [unwired: 8 in, 1 out]
            n87 = call <vilib>:"Add State(s) to Queue__jki_lib_state_machine.vi"("State(s) in (\"\")"=w274) -> ("States Out"=w273:string)  [unwired: 14 in]
          }
          frame "Events: Register" {
            # "Expand to add\nmore events"
            # "Self Events (API Calls)"
            # "Base Class Protected Events"
            n88 = Unbundle By Name(w282) -> ("Self Reference"=w279:refnum<class "SystemController.lvclass">)
            n89 = call <vilib>:"GetProtectedEvents.vi"("SMO"=w279) -> ("error out"=w276:errorcluster, "SMO Protected Events"=w280:T12)  [unwired: 8 in, 1 out]
            n90 = register-events(w280) -> (reference out=w281:refnum<event-registration>, error out=w277:errorcluster)  [unwired: 2 in]
            n91 = Merge Errors(w278, w277, w276) -> (w275:errorcluster)
            n92 = call <vilib>:"Add State(s) to Queue__jki_lib_state_machine.vi"("State(s) in (\"\")"=w284) -> ("States Out"=w283:string)  [unwired: 14 in]
          }
          frame "Events: Unregister" {
            n93 = Unregister For Events(event registration refnum=w287, error in=w286) -> (error out=w285:errorcluster)
            n94 = call <vilib>:"Clear Errors.vi"("error in (no error)"=w285) -> ()  [unwired: 5 in, 2 out]
            n95 = call <vilib>:"Add State(s) to Queue__jki_lib_state_machine.vi"("State(s) in (\"\")"=w290) -> ("States Out"=w289:string)  [unwired: 14 in]
          }
          frame "---------- Camera ----------" {
            n96 = call <vilib>:"Add State(s) to Queue__jki_lib_state_machine.vi"("State(s) in (\"\")"=w295) -> ("States Out"=w294:string)  [unwired: 14 in]
          }
          frame "Camera: Connect" {
            n97 = Unbundle By Name(w299) -> ("Dependencies.Camera"=w298:refnum<class "Camera.lvclass">)
            n98 = call-dynamic "Connect.vi"("error in (no error)"=w297, "reference in"=w298) -> ("error out"=w296:errorcluster)  [unwired: 8 in, 1 out]
            n99 = call <vilib>:"Add State(s) to Queue__jki_lib_state_machine.vi"("State(s) in (\"\")"=w302) -> ("States Out"=w301:string)  [unwired: 14 in]
          }
          frame "Camera: Disconnect" {
            n100 = Unbundle By Name(w306) -> ("Dependencies.Camera"=w305:refnum<class "Camera.lvclass">)
            n101 = call-dynamic "Disconnect.vi"("error in (no error)"=w304, "reference in"=w305) -> ("error out"=w303:errorcluster)  [unwired: 8 in, 1 out]
            n102 = call <vilib>:"Add State(s) to Queue__jki_lib_state_machine.vi"("State(s) in (\"\")"=w309) -> ("States Out"=w308:string)  [unwired: 14 in]
          }
          frame "Camera: Start Acquisition" {
            n103 = Unbundle By Name(w313) -> ("Dependencies.Camera"=w312:refnum<class "Camera.lvclass">)
            n104 = call-dynamic "StartAcquisition.vi"("error in (no error)"=w311, "reference in"=w312) -> ("error out"=w310:errorcluster)  [unwired: 8 in, 1 out]
            n105 = call <vilib>:"Add State(s) to Queue__jki_lib_state_machine.vi"("State(s) in (\"\")"=w316) -> ("States Out"=w315:string)  [unwired: 14 in]
          }
          frame "Camera: Stop Acquisition" {
            n106 = Unbundle By Name(w320) -> ("Dependencies.Camera"=w319:refnum<class "Camera.lvclass">)
            n107 = call-dynamic "StopAcquisition.vi"("error in (no error)"=w318, "reference in"=w319) -> ("error out"=w317:errorcluster)  [unwired: 8 in, 1 out]
            n108 = call <vilib>:"Add State(s) to Queue__jki_lib_state_machine.vi"("State(s) in (\"\")"=w323) -> ("States Out"=w322:string)  [unwired: 14 in]
          }
          frame "Camera: Grab" {
            n109 = Unbundle By Name(w330) -> ("Dependencies.Camera"=w332:refnum<class "Camera.lvclass">, "New Image"=w327:T1)
            n110 = call-dynamic "Grab.vi"("error in (no error)"=w331, "reference in"=w332) -> ("error out"=w325:errorcluster, "Image Out"=w328:T1)  [unwired: 6 in, 2 out]
            n111 = call "IMAQ Copy"("error in (no error)"=w325, "Image Dst"=w327, "Image Src"=w328) -> ("error out"=w324:errorcluster, "Image Dst Out"=w326:T1)  [unwired: 3 in]
            n112 = Bundle By Name(cluster=w330, "New Image"=w326) -> (w329:T10)
            n113 = call <vilib>:"Add State(s) to Queue__jki_lib_state_machine.vi"("State(s) in (\"\")"=w335) -> ("States Out"=w334:string)  [unwired: 14 in]
          }
          frame "Camera: Get Connected" {
            n114 = Unbundle By Name(w338) -> ("Dependencies.Camera"=w341:refnum<class "Camera.lvclass">)
            n115 = call-dynamic "GetConnected.vi"("error in (no error)"=w340, "reference in"=w341) -> ("error out"=w339:errorcluster, "Connected"=w336:bool)  [unwired: 7 in, 1 out]
            "Connected" <- w336
            n116 = Bundle By Name(cluster=w338, "Camera Connected"=w336) -> (w337:T10)
            n117 = call <vilib>:"Add State(s) to Queue__jki_lib_state_machine.vi"("State(s) in (\"\")"=w344) -> ("States Out"=w343:string)  [unwired: 14 in]
          }
          frame "---------- Facial Recognition ----------" {
            n118 = call <vilib>:"Add State(s) to Queue__jki_lib_state_machine.vi"("State(s) in (\"\")"=w349) -> ("States Out"=w348:string)  [unwired: 14 in]
          }
          frame "Facial Recognition: Find Faces" {
            n119 = Unbundle By Name(w352) -> ("Dependencies.ImageFacialDetection"=w356:refnum<class "ImageFacialDetection.lvclass">, "New Image"=w355:T1)
            n120 = call-poly "FindFaces.vi"("error in (no error)"=w354, "image"=w355, "reference in"=w356) -> ("error out"=w353:errorcluster, "image with faces"=w350:T1)  [unwired: 6 in, 1 out]
            n121 = Bundle By Name(cluster=w352, "New Image"=w350) -> (w351:T10)
            n122 = call <vilib>:"Add State(s) to Queue__jki_lib_state_machine.vi"("State(s) in (\"\")"=w359) -> ("States Out"=w358:string)  [unwired: 14 in]
          }
          frame "Facial Recognition: Find Eyes" {
            n123 = Unbundle By Name(w362) -> ("Dependencies.ImageFacialDetection"=w366:refnum<class "ImageFacialDetection.lvclass">, "New Image"=w365:T1)
            n124 = call-poly "FindEyes.vi"("error in (no error)"=w364, "image"=w365, "reference in"=w366) -> ("error out"=w363:errorcluster, "image with faces"=w360:T1)  [unwired: 6 in, 1 out]
            n125 = Bundle By Name(cluster=w362, "New Image"=w360) -> (w361:T10)
            n126 = call <vilib>:"Add State(s) to Queue__jki_lib_state_machine.vi"("State(s) in (\"\")"=w369) -> ("States Out"=w368:string)  [unwired: 14 in]
          }
          frame "---------- Image ----------" {
            n127 = call <vilib>:"Add State(s) to Queue__jki_lib_state_machine.vi"("State(s) in (\"\")"=w374) -> ("States Out"=w373:string)  [unwired: 14 in]
          }
          frame "Image: Set" {
            n128 = Unbundle By Name(w379) -> ("Self Reference"=w378:refnum<class "SystemController.lvclass">, "New Image"=w375:T1)
            "Image" <- w375
            n129 = call "SystemController.SetImage.vi"("error in (no error)"=w377, "Image"=w375, "SystemController"=w378) -> ("error out"=w376:errorcluster)  [unwired: 7 in, 1 out]
            n130 = call <vilib>:"Add State(s) to Queue__jki_lib_state_machine.vi"("State(s) in (\"\")"=w382) -> ("States Out"=w381:string)  [unwired: 14 in]
          }
        }
      }
    }
    frame Error {
    }
  }
  n131 = call-parent "Process.vi"("error in"=w7, "SMO"=w6) -> ("error out"=w4:errorcluster, "SMO out"=→"SystemController out":refnum<class "SystemController.lvclass">)  [unwired: 8 in]
  n132 = Merge Errors(w4, w3) -> (→"error out":errorcluster)
